vi "stage read_v2.vi"(3 "Axis":u32, 4 "Incoming Handle":i32, 5 "read #":i32=7) -> (0 "Outgoing Handle":i32, 1 "position (um)":dbl)   [LabVIEW 2014]
uses:
  <vilib>/Analysis/baseanly.llb/Mean (DBL).vi
  <vilib>/Analysis/NI_AALBase.lvlib
  MCL-dll-Labview 32-bit/Madlib.dll
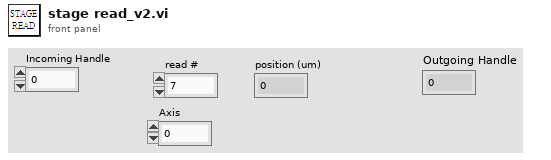
[diagram p1: front panel]
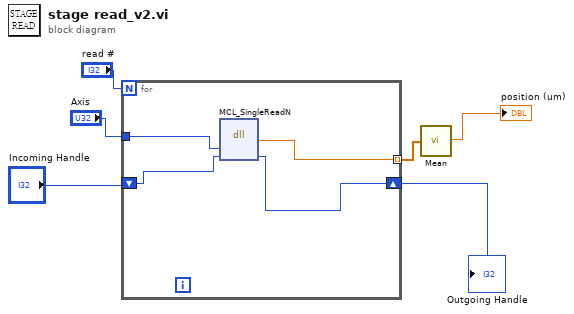
[diagram p0: block diagram]
diagram:
  n1 = for {
    N: "read #" -> [_]
    tunnel: "Axis" -> [w10]
    tunnel: [w9] -> w4 mode=indexing
    shift-right: [w8] -> w1
    shift-left: "Incoming Handle" -> [w7]
    n2 = dll-call lib="C:/Users/OT-hwlab/Desktop/YCC's OT/Main/Main-Stage-Based/SubVI-Stage-Based/MCL-dll-Labview 32-bit/Madlib.dll" fn="MCL_SingleReadN"("axis"=w10, "handle"=w7) -> ("return type"=w9:dbl, "handle"=w8:i32)  [unwired: 4 in, 2 out]
  }
  "Outgoing Handle" <- w1
  n3 = call-poly <vilib>:"Mean.vi"("X"=w4) -> ("mean"=→"position (um)":dbl)  [unwired: 1 out]
